vi "Query Instrument Status.vi"(8 "error in (no error)":errorcluster, 10 "Instrument Status (0: Standard Event Status Enable Register)":u32(ring) items=["Standard Event Status Enable Register", "Service Request Enable Register", "Status Byte Register", "Standard Event Status Register"], 11 "VISA resource name":refnum<visa-resource-name>) -> (0 "error out":errorcluster, 2 "Register Value":u32, 3 "VISA resource name out":refnum<visa-resource-name>)   [LabVIEW 2022 SP3, in "MagnaDC.lvlib"]
uses:
  MagnaDC.lvlib
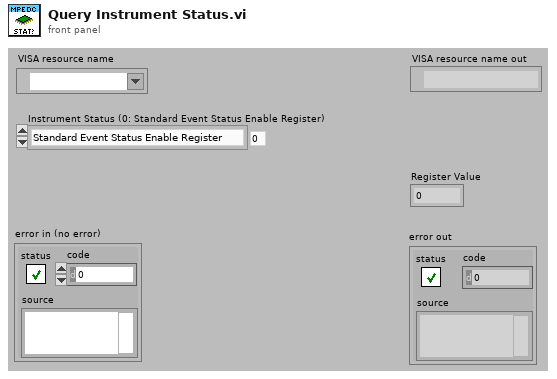
[diagram p1: front panel]
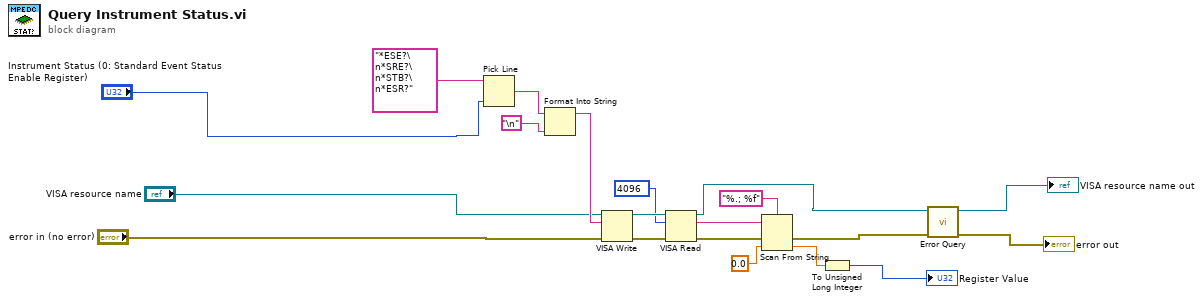
[diagram p0: block diagram]
diagram:
  n1 = Pick Line(multi-line string="*ESE?\n*SRE?\n*STB?\n*ESR?", line index="Instrument Status (0: Standard Event Status Enable Register)") -> (output string=w9:string)  [unwired: 1 in]
  n2 = Format Into String(initial string=w9, "\n") -> (resulting string=w8:string)  [unwired: 2 in, 1 out]
  n3 = VISA Write(VISA resource name="VISA resource name", write buffer=w8, error in (no error)="error in (no error)") -> (VISA resource name out=w18:refnum<visa-resource-name>, error out=w17:errorcluster)  [unwired: 1 out]
  n4 = VISA Read(VISA resource name=w18, byte count=u32 4096, error in (no error)=w17) -> (VISA resource name out=w6:refnum<visa-resource-name>, read buffer=w15:string, error out=w13:errorcluster)  [unwired: 1 out]
  n5 = Scan From String(format string="%.; %f", input string=w15, error in=w13, default 1=0.0 ("default value 1")) -> (error out=w5:errorcluster, output 1=w7:dbl)  [unwired: 1 in, 2 out]
  n6 = To Unsigned Long Integer(number=w7) -> (unsigned 32bit integer=→"Register Value":u32)
  n7 = call "Error Query.vi"("error in (no error)"=w5, "VISA resource name"=w6) -> ("error out"=→"error out":errorcluster, "VISA resource name out"=→"VISA resource name out":refnum<visa-resource-name>)  [unwired: 6 in, 2 out]
